vi "Build Feed.vi"(0 "Packages Path":path, 11 "error in (no error)":errorcluster) -> (15 "error out":errorcluster)   [LabVIEW 2021, in "Packager Helpers.lvlib"]
uses:
  Packager Helpers.lvlib
  Path Functions/Path Functions.lvlib
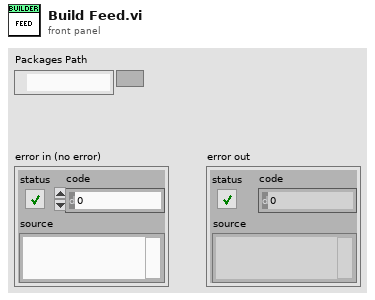
[diagram p1: front panel]
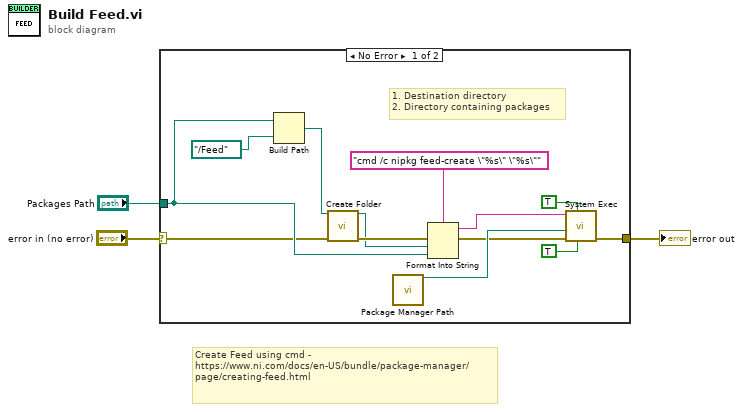
[diagram p0: block diagram]
diagram:
  # "Create Feed using cmd -\nhttps://www.ni.com/docs/en-US/bundle/package-manager/page/creating-feed.html"
  n1 = case shown="No Error" "error in (no error)" {
    selector: "error in (no error)" -> [w11 w17]
    tunnel: "Packages Path" -> [w14 _]
    tunnel: [w4 w17] -> w1
    frame No Error {
      # "1. Destination directory\n2. Directory containing packages"
      n2 = Build Path(base path=w14, name or relative path=path "../Feed") -> (appended path=w12:path)
      n3 = call "Create Folder.vi"("Directory Path"=w12, "error in (no error)"=w11) -> ("Dup Directory Path"=w9:path, "error out"=w10:errorcluster)  [unwired: 12 in]
      n4 = call "Package Manager Path.vi"() -> ("Package Manager Path"=w16:path)  [unwired: 15 in]
      n5 = Format Into String(format string="cmd /c nipkg feed-create \"%s\" \"%s\"", error in=w10, w9, w14) -> (resulting string=w7:string, error out=w8:errorcluster)  [unwired: 1 in]
      n6 = call <vilib>:"System Exec.vi"("run minimized? (F)"=TRUE, "wait until completion? (T)"=TRUE, "error in (no error)"=w8, "working directory"=w16, "command line"=w7) -> ("error out"=w4:errorcluster)  [unwired: 3 in, 3 out]
    }
    frame Error {
    }
  }
  "error out" <- w1
